vi "SE FP behavior S-Wall.vi"(1 "Behavior\nVelocity":dbl, 2 "Activate?":bool=TRUE, 3 "IR Sensors":T1(array[cluster])) -> (0 "S-Wall Array":dbl[](array[numeric]))   [LabVIEW 2014]
panel:
  out "Waveform Graph":cluster{dbl, dbl, dbl[]}(graph)
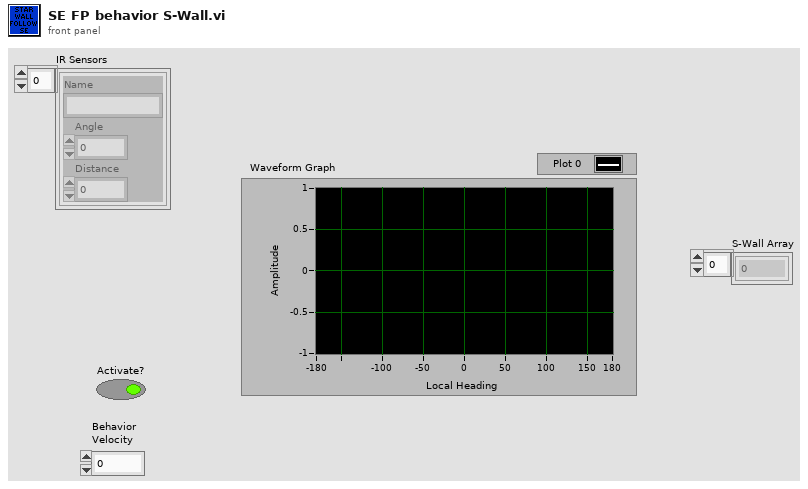
[diagram p1: front panel]
types:
  T1 = cluster{"Name":string, "Angle":dbl, "Distance":dbl}[]
  T2 = cluster{"Name":string, "Angle":dbl, "Distance":dbl}
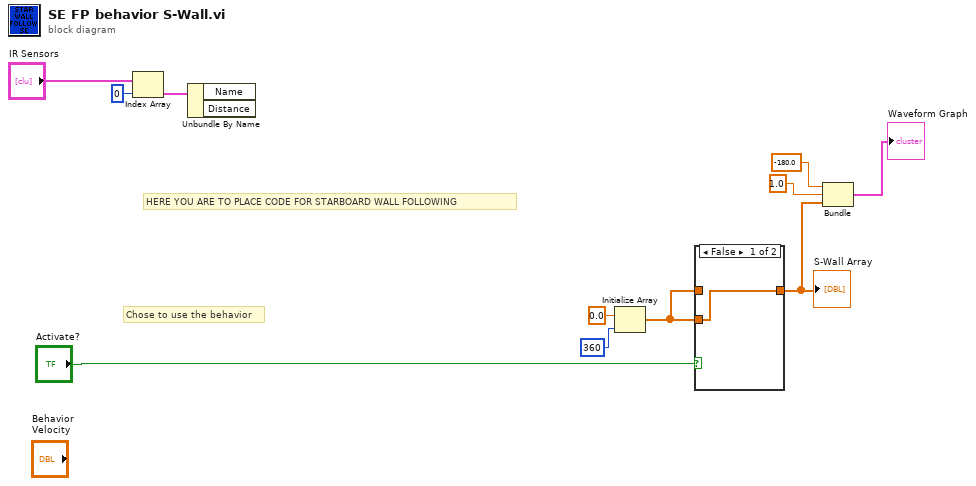
[diagram p0: block diagram]
diagram:
  # "HERE YOU ARE TO PLACE CODE FOR STARBOARD WALL FOLLOWING"
  # "Chose to use the behavior"
  n1 = Index Array(array="IR Sensors", index=0) -> (element=w10:T2)
  n2 = Unbundle By Name(w10) -> ()  [unwired: 2 out]
  n3 = Initialize Array(0.0 ("element"), 360 ("dimension size")) -> (w3:dbl[])
  n4 = case shown="False" "Activate?" {
    tunnel: w3 -> [w12 _]
    tunnel: w3 -> [_ w13]
    tunnel: [w12 w13] -> w2
    frame False {
    }
    frame True {
    }
  }
  "S-Wall Array" <- w2
  n5 = Bundle(-180.0, 1.0, w2) -> (→"Waveform Graph":cluster{dbl, dbl, dbl[]})  [unwired: 1 in]
